vi "simpleDLL.vi"() -> ()   [LabVIEW 2015]
uses:
  SimpleDLLSecond.lvlib
panel:
  in  "Tab Control":enum32{"Page 1"}(tab)
  in  "Multiply":bool
  in  "Divide":bool
  in  "Substract":bool
  in  "Add":bool
  out "function return":dbl
  in  "stop":bool
  in  "a":dbl
  in  "b":dbl
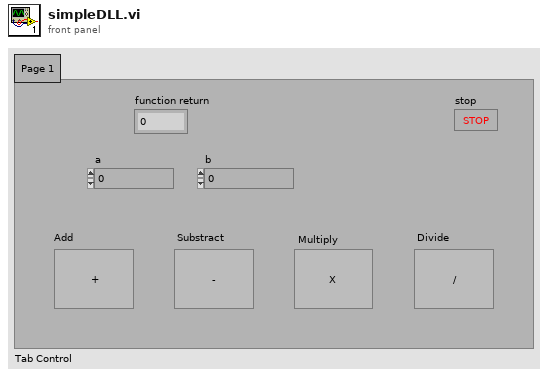
[diagram p1: front panel]
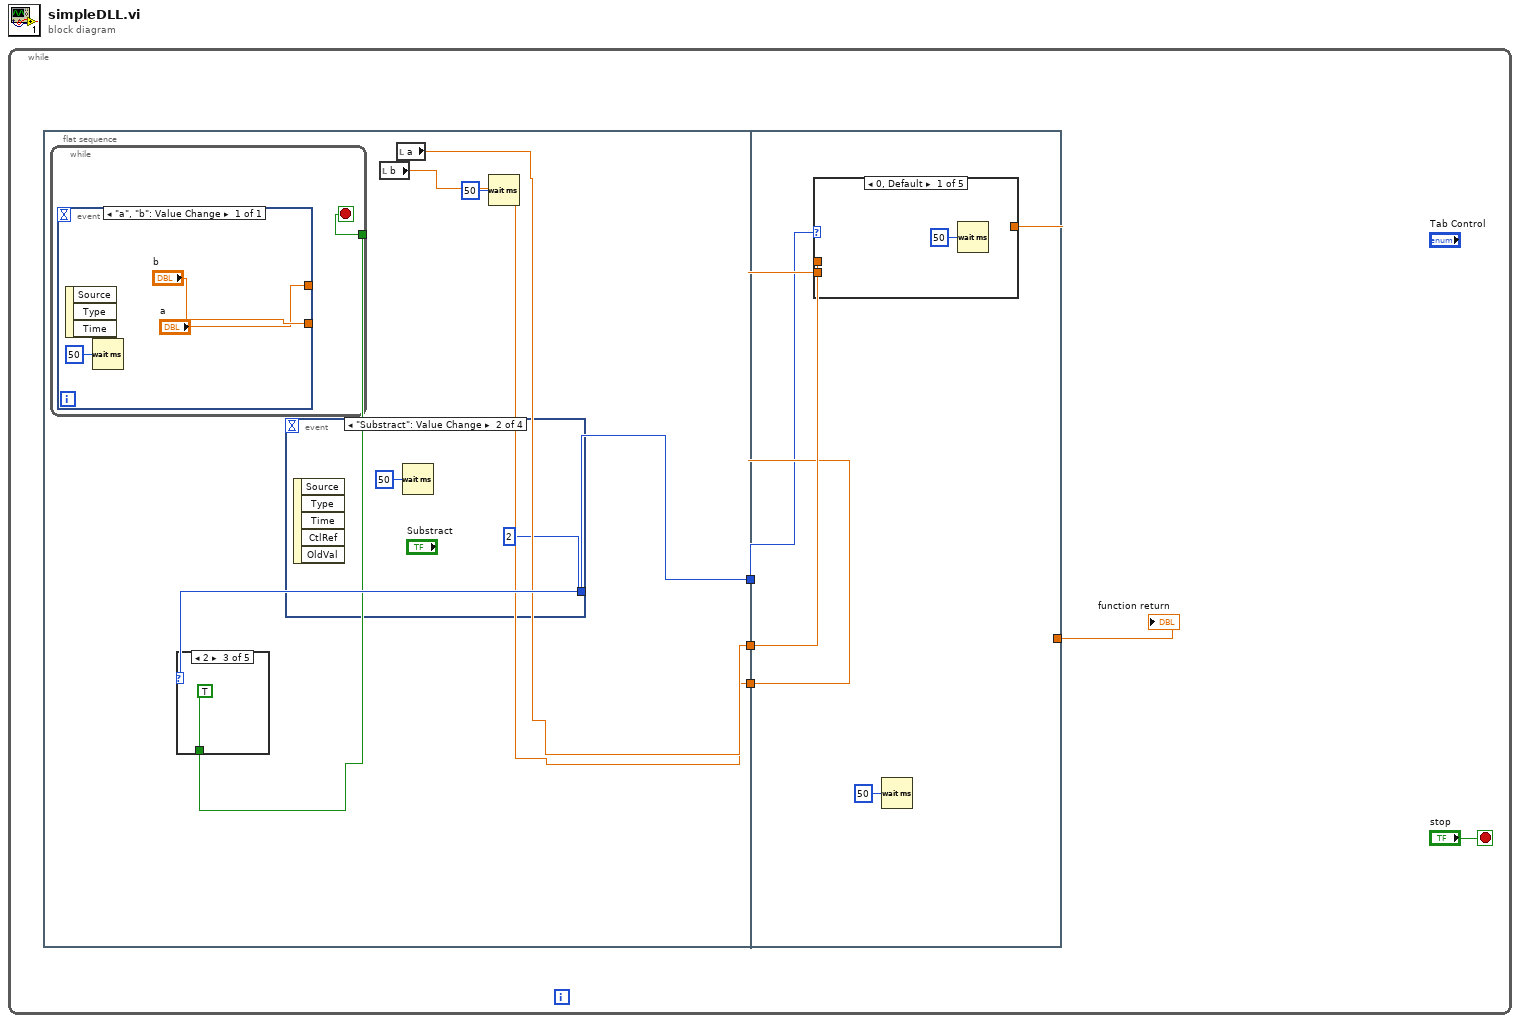
[diagram p0: block diagram]
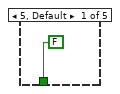
[diagram p2: hidden frame]
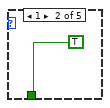
[diagram p3: hidden frame]
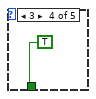
[diagram p4: hidden frame]
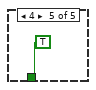
[diagram p5: hidden frame]
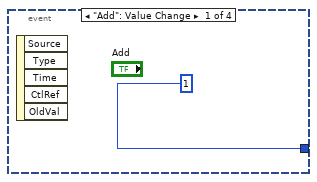
[diagram p6: hidden frame]
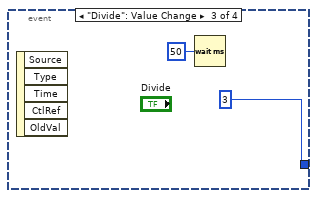
[diagram p7: hidden frame]
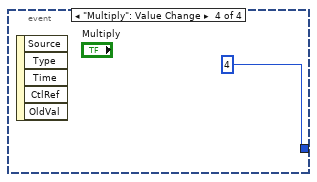
[diagram p8: hidden frame]
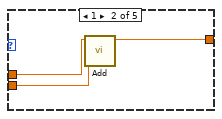
[diagram p9: hidden frame]
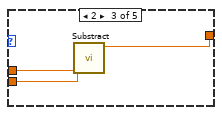
[diagram p10: hidden frame]
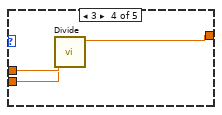
[diagram p11: hidden frame]
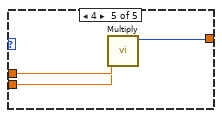
[diagram p12: hidden frame]
diagram:
  n1 = while {
    stop <- "stop" stop-if-true
    n2 = flat-sequence {
      tunnel: [w7] -> w3
      tunnel: [w6] -> w2
      tunnel: [w10] -> w1
      tunnel: [w30] -> w4
      tunnel: w3 -> [w29]
      tunnel: w2 -> [w28]
      tunnel: w1 -> [w27]
      frame #0 {
        n3 = event shown="[1] \"Substract\": Value Change" {
          selector: _ -> [_ _ _ _]
          dyn-events: _ -> [_ _ _ _]
          timeout: _ -> [_ _ _ _]
          tunnel: [1 2 3 4] -> w10
          event "Add": Value Change {
            n4 = event-data() -> ()  [unwired: 1 in, 5 out]
          }
          event "Substract": Value Change {
            n5 = event-data() -> ()  [unwired: 1 in, 5 out]
            n6 = Wait (ms)(milliseconds to wait=u32 50) -> ()  [unwired: 1 out]
          }
          event "Divide": Value Change {
            n7 = event-data() -> ()  [unwired: 1 in, 5 out]
            n8 = Wait (ms)(milliseconds to wait=u32 50) -> ()  [unwired: 1 out]
          }
          event "Multiply": Value Change {
            n9 = event-data() -> ()  [unwired: 1 in, 5 out]
          }
        }
        n10 = case shown="2" w10 {
          tunnel: [FALSE TRUE TRUE TRUE TRUE] -> w8
          frame 5, Default {
          }
          frame 1 {
          }
          frame 2 {
          }
          frame 3 {
          }
          frame 4 {
          }
        }
        n11 = while {
          tunnel: w8 -> [w11]
          stop <- w11 stop-if-true
          n12 = event shown="[0] \"a\", \"b\": Value Change" {
            selector: _ -> [_]
            dyn-events: _ -> [_]
            timeout: _ -> [_]
            tunnel: ["a"] -> _
            tunnel: ["b"] -> _
            event "a", "b": Value Change {
              n13 = event-data() -> ()  [unwired: 1 in, 3 out]
              n14 = Wait (ms)(milliseconds to wait=u32 50) -> ()  [unwired: 1 out]
            }
          }
        }
        n15 = local read "b"() -> (w6:dbl)
        n16 = local read "a"() -> (w7:dbl)
        n17 = Wait (ms)(milliseconds to wait=u32 50) -> ()  [unwired: 1 out]
      }
      frame #1 {
        n18 = case shown="0, Default" w27 {
          tunnel: [_ w34 w37 w40 w43] -> w30
          tunnel: w29 -> [_ w33 w36 w39 w42]
          tunnel: w28 -> [_ w32 w35 w38 w41]
          frame 0, Default {
            n19 = Wait (ms)(milliseconds to wait=u32 50) -> ()  [unwired: 1 out]
          }
          frame 1 {
            n20 = call "Add.vi"("d"=w32, "c"=w33) -> ("function return"=w34:dbl)  [unwired: 9 in]
          }
          frame 2 {
            n21 = call "Substract.vi"("d"=w35, "c"=w36) -> ("function return"=w37:dbl)  [unwired: 9 in]
          }
          frame 3 {
            n22 = call "Divide.vi"("d"=w38, "c"=w39) -> ("function return"=w40:dbl)  [unwired: 9 in]
          }
          frame 4 {
            n23 = call "Multiply.vi"("d"=w41, "c"=w42) -> ("function return"=w43:i32)  [unwired: 9 in]
          }
        }
        n24 = Wait (ms)(milliseconds to wait=u32 50) -> ()  [unwired: 1 out]
      }
    }
    "function return" <- w4
  }
